vi "Sweep Actions.vi"(0 "VISA resource name":refnum<visa-resource-name>, 5 "Sweep (0:Continuous Measurement)":i32(ring) items=["Continuous Measurement", "Single Measurement", "Single Sweep", "Stop Sweep", "Restart Sweep", "Linear Average Sweep", "Average Sweep", "Max Hold Sweep", "Min Hold Sweep"], 11 "error in (no error)":errorcluster) -> (4 "VISA resource name out":refnum<visa-resource-name>, 15 "error out":errorcluster)   [LabVIEW 2020, in "Anritsu Signal Analyzer Series.lvlib"]
doc: "Sets the Sweep Action.\n\nSets the sweep mode to Continuous and starts continuous sweep.\nSets the sweep mode to Single and start the single sweep.\nSets the sweep mode to single and starts single sweep. Also, reads sweep status (End sweep/Sweeping).\nSets the sweep mode to Stops sweep.\nSets the sweep mode to Restarts sweep.\nSets storage mode to linear average and starts sweep.\nSets the storage mode to average and starts sweep.\nSets the storage mode to Max Hold and start sweep.\nSets the storage mode to Max Hold and start sweep."
uses:
  Anritsu Signal Analyzer Series.lvlib
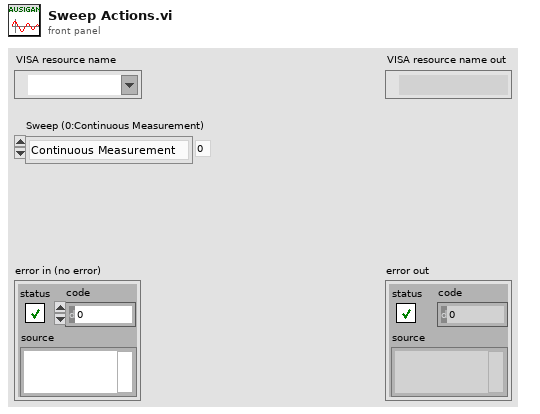
[diagram p1: front panel]
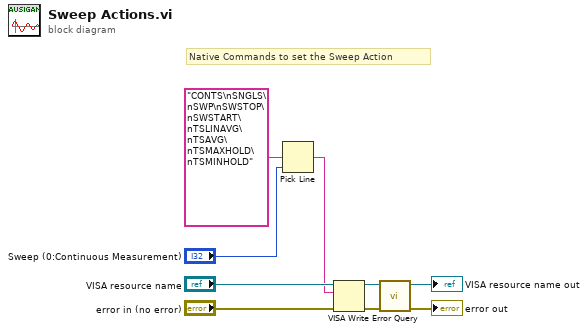
[diagram p0: block diagram]
diagram:
  # "Native Commands to set the Sweep Action"
  n1 = Pick Line(multi-line string="CONTS\nSNGLS\nSWP\nSWSTOP\nSWSTART\nTSLINAVG\nTSAVG\nTSMAXHOLD\nTSMINHOLD" ("_Command"), line index="Sweep (0:Continuous Measurement)") -> (output string=w3:string)  [unwired: 1 in]
  n2 = VISA Write(VISA resource name="VISA resource name", write buffer=w3, error in (no error)="error in (no error)") -> (VISA resource name out=w2:refnum<visa-resource-name>, error out=w1:errorcluster)  [unwired: 1 out]
  n3 = call "Error Query.vi"("error in (no error)"=w1, "VISA resource name"=w2) -> ("error out"=→"error out":errorcluster, "VISA resource name out"=→"VISA resource name out":refnum<visa-resource-name>)  [unwired: 6 in, 2 out]
